vi "LPC set transmission.vi"(8 "error in (no error)":errorcluster, 10 "transmission (%)":dbl=75.0, 11 "VISA resource name":refnum<visa-resource-name>="GPIB0::8::INSTR") -> (0 "error out":errorcluster, 3 "VISA resource name out":refnum<visa-resource-name>)   [LabVIEW 2015, in "BEOC LPC.lvlib"]
doc: "Sets the transmission of the LPC (laser power controller)."
uses:
  BEOC LPC.lvlib
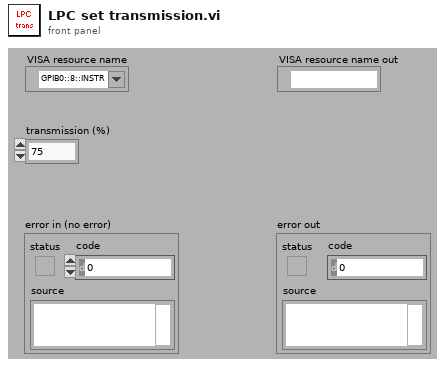
[diagram p1: front panel]
types:
  T1 = typedef "Semaphore RefNum" = refnum<k1>
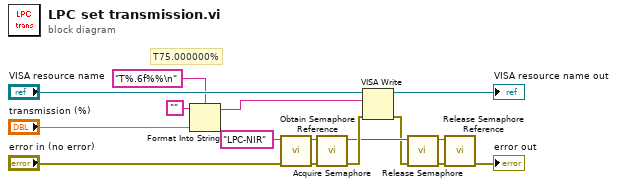
[diagram p0: block diagram]
diagram:
  # "T75.000000%"
  n1 = Format Into String(format string="T%.6f%%\n", initial string="", "transmission (%)") -> (resulting string=w12:string)  [unwired: 1 in, 1 out]
  n2 = call <vilib>:"Obtain Semaphore Reference.vi"("error in (no error)"="error in (no error)", "name (unnamed)"="LPC-NIR") -> ("error out"=w7:errorcluster, "semaphore"=w6:T1)  [unwired: 1 in, 3 out]
  n3 = call <vilib>:"Acquire Semaphore.vi"("error in (no error)"=w7, "semaphore"=w6) -> ("error out"=w3:errorcluster, "semaphore out"=w2:T1)  [unwired: 1 in, 3 out]
  n4 = VISA Write(VISA resource name="VISA resource name", write buffer=w12, error in (no error)=w3) -> (VISA resource name out=→"VISA resource name out":refnum<visa-resource-name>, error out=w1:errorcluster)  [unwired: 1 out]
  n5 = call <vilib>:"Release Semaphore.vi"("error in (no error)"=w1, "semaphore"=w2) -> ("error out"=w5:errorcluster, "semaphore out"=w4:T1)  [unwired: 4 out]
  n6 = call <vilib>:"Release Semaphore Reference.vi"("error in (no error)"=w5, "semaphore"=w4) -> ("error out"=→"error out":errorcluster)  [unwired: 9 out]
